vi "libreply.vi"(8 "error in (no error)":errorcluster, 9 "parameter":string, 10 "id":string, 11 "output":i32) -> (0 "error out":errorcluster)   [LabVIEW 2015]
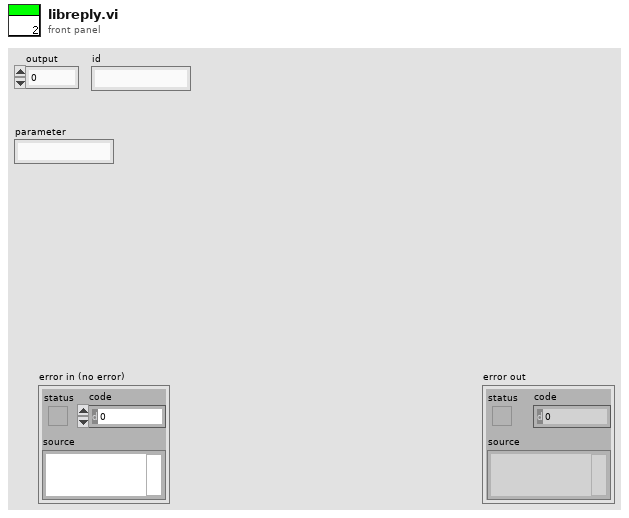
[diagram p1: front panel]
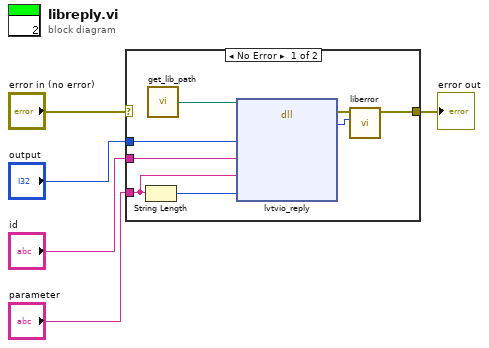
[diagram p0: block diagram]
diagram:
  n1 = case shown="No Error" "error in (no error)" {
    selector: "error in (no error)" -> [_ w14]
    tunnel: [w6 w14] -> w4
    tunnel: "parameter" -> [w11 _]
    tunnel: "id" -> [w10 _]
    tunnel: "output" -> [w9 _]
    frame No Error {
      n2 = String Length(string=w11) -> (length=w12:i32)
      n3 = call "get_lib_path.vi"() -> ("Path"=w13:path)
      n4 = dll-call lib="S:/thingiverselv/lib/liblvtvio.dll" fn="lvtvio_reply"(path in=w13, "output"=w9, "id"=w10, "params"=w11, "params_size"=w12) -> (error out=w8:errorcluster, "return type"=w7:i32)  [unwired: 6 in, 1 out]
      n5 = call "liberror.vi"("tvio errors"=w7, "error in (no error)"=w8) -> ("error out"=w6:errorcluster)  [unwired: 9 in]
    }
    frame Error {
    }
  }
  "error out" <- w4
